vi "稱號-骰子賭聖.vi"() -> ()   [LabVIEW 2014]
panel:
  in  "退出視窗":bool
  # "恭喜獲得稱號:"
  # "代表你在骰子方面的賭運很好，但要記住不可沉迷過深喔!"
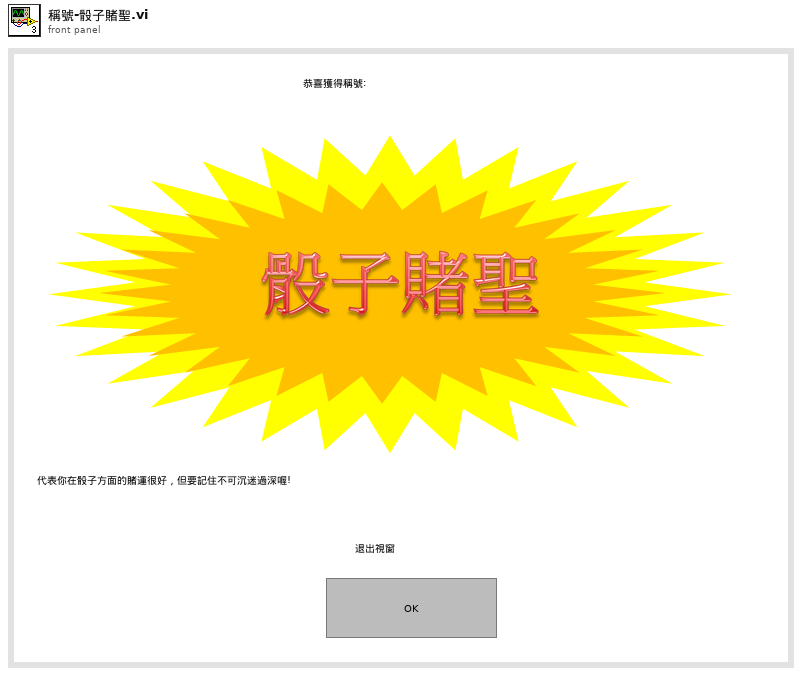
[diagram p1: front panel]
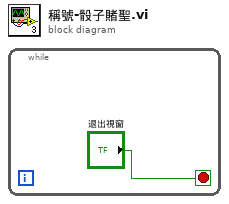
[diagram p0: block diagram]
diagram:
  n1 = while {
    stop <- "退出視窗" stop-if-true
  }
